vi "Freefield-Compute ASTF.vi"(0 "Stimulus":dbl[](array[numeric]), 5 "Response":dbl[](array[numeric]), 7 "Fs (Hz)":dbl=1.0, 9 "Response params":T2, 11 "error in (no error)":errorcluster) -> (6 "data":T1, 15 "error out":errorcluster)   [LabVIEW 2020]
uses:
  Common VIs/Typedefs/CAL-Response.ctl
  Common VIs/Typedefs/CAL-Data.ctl
  epl-vi-lib/Utility VIs/Math VIs/FFT x(t) to dB,Degrees (1D).vi
panel:
  out "Frequency":dbl[](array[numeric])
  out "ASTF Phase":dbl[](array[numeric])
  out "ASTF Mag":dbl[](array[numeric])
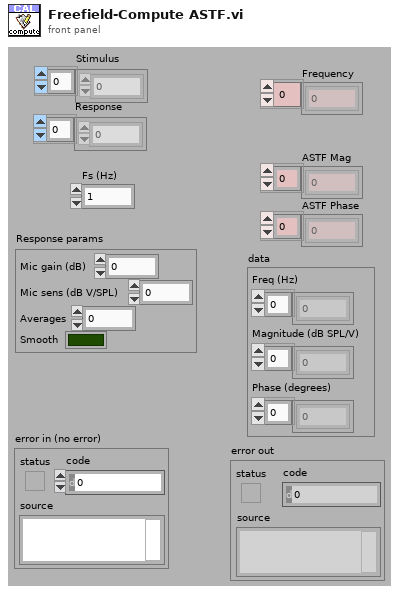
[diagram p1: front panel]
types:
  T1 = typedef "CAL-Data.ctl" = cluster{"Freq (Hz)":dbl[], "Magnitude (dB SPL/V)":dbl[], "Phase (degrees)":dbl[]}
  T2 = typedef "CAL-Response.ctl" = cluster{"Mic gain (dB)":dbl, "Mic sens (dB V/SPL)":dbl, "Averages":i32, "Smooth":bool}
  T3 = cluster{"Freq (Hz)":dbl[], "Magnitude Smoothed":dbl[], dbl[]}
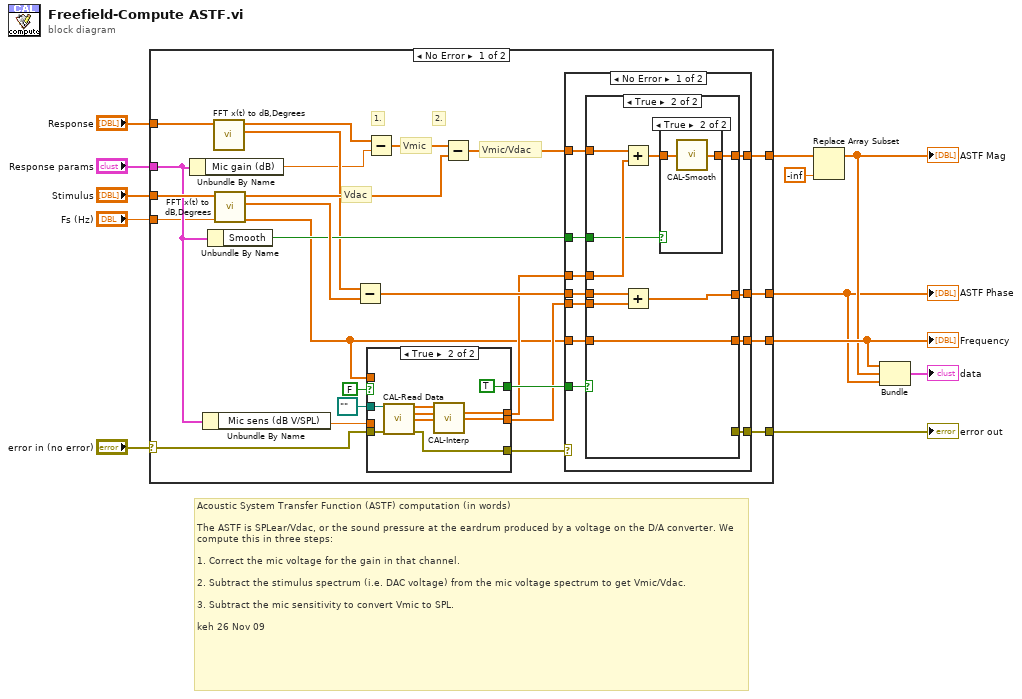
[diagram p0: block diagram]
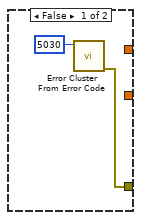
[diagram p2: hidden frame]
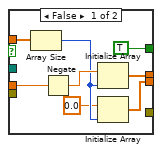
[diagram p5: hidden frame]
diagram:
  # "Acoustic System Transfer Function (ASTF) computation (in words)\n\nThe ASTF is SPLear/Vdac, or the sound pressure at the eardrum produced by a voltage on the D/A converter. We compute this in three steps:\n\n1. Correct the mic voltage for the gain in that channel.\n\n2. Subtract the stimulus spectrum (i.e. DAC voltage) from the mic voltage spectrum to get Vmic/Vdac.\n\n3. Subtract the mic sensitivity to convert Vmic to SPL.\n\nkeh 26 Nov 09"
  n1 = case shown="No Error" "error in (no error)" {
    selector: "error in (no error)" -> [w32 w82]
    tunnel: "Response" -> [w19 _]
    tunnel: [w35 _] -> w11
    tunnel: [w28 _] -> w2
    tunnel: "Stimulus" -> [w38 _]
    tunnel: [w24 _] -> w4
    tunnel: [w25 w82] -> w8
    tunnel: "Response params" -> [w14 _]
    tunnel: "Fs (Hz)" -> [w13 _]
    frame No Error {
      # "2."
      # "1."
      # "Vmic/Vdac"
      # "Vdac"
      # "Vmic"
      n2 = Unbundle By Name(w14) -> ("Mic gain (dB)"=w15:dbl)
      n3 = Unbundle By Name(w14) -> ("Mic sens (dB V/SPL)"=w31:dbl)
      n4 = Unbundle By Name(w14) -> ("Smooth"=w22:bool)
      n5 = call-poly "FFT x(t) to dB,Degrees.vi"("X"=w19) -> ("+Freq Phase of FFT (degrees)"=w17:dbl[], "+Freq. Mag of FFT (dB rms)"=w18:dbl[])  [unwired: 8 in, 1 out]
      n6 = call-poly "FFT x(t) to dB,Degrees.vi"("Fs (Hz)"=w13, "X"=w38) -> ("Freq (Hz)"=w16:dbl[], "+Freq Phase of FFT (degrees)"=w37:dbl[], "+Freq. Mag of FFT (dB rms)"=w36:dbl[])  [unwired: 7 in]
      n7 = Subtract(x=w17, y=w37) -> (x-y=w29:dbl[])
      n8 = Subtract(x=w18, y=w15) -> (x-y=w34:dbl[])
      n9 = case shown="True" FALSE {
        tunnel: w32 -> [_ w81]
        tunnel: w16 -> [w72 _]
        tunnel: path "" ("Path") -> [_ w80]
        tunnel: w31 -> [w71 _]
        tunnel: [TRUE ("arrays equal?") TRUE ("arrays equal?")] -> w27
        tunnel: [_ w79] -> w30
        tunnel: [w70 w75] -> w26
        tunnel: [w66 w74] -> w23
        frame False {
          n10 = Array Size(array=w72) -> (size(s)=w68:i32)
          n11 = Negate(x=w71) -> (-x=w69:dbl)
          n12 = Initialize Array(w69, w68) -> (w70:dbl[])
          n13 = Initialize Array(0.0 ("element"), w68) -> (w66:dbl[])
        }
        frame True {
          n14 = call "CAL-Read Data.vi"("user path"=w80, "error in (no error)"=w81) -> ("Frequency (Hz)"=w78:dbl[], "Mag"=w77:dbl[], "Phase"=w76:dbl[], "error out"=w79:errorcluster)  [unwired: 9 in, 1 out]
          n15 = call "CAL-Interp.vi"("Frequency (Hz)"=w78, "Magnitude (dB)"=w77, "Phase (degrees)"=w76) -> ("Interp Magnitude (dB)"=w75:dbl[], "Interp Phase (degrees)"=w74:dbl[])  [unwired: 9 in, 2 out]
        }
      }
      n16 = Subtract(x=w34, y=w36) -> (x-y=w33:dbl[])
      n17 = case shown="No Error" w30 {
        selector: w30 -> [_ w64]
        tunnel: w26 -> [w49 _]
        tunnel: [w48 _] -> w35
        tunnel: w33 -> [w47 _]
        tunnel: [w43 w64] -> w25
        tunnel: w29 -> [w45 _]
        tunnel: [w44 _] -> w28
        tunnel: w27 -> [w46 _]
        tunnel: w16 -> [w42 _]
        tunnel: [w41 _] -> w24
        tunnel: w23 -> [w40 _]
        tunnel: w22 -> [w39 _]
        frame No Error {
          n18 = case shown="True" w46 {
            tunnel: w49 -> [_ w60]
            tunnel: [_ w52] -> w48
            tunnel: w47 -> [_ w59]
            tunnel: w45 -> [_ w58]
            tunnel: [_ w57] -> w44
            tunnel: [w51 _] -> w43
            tunnel: w42 -> [_ w56]
            tunnel: [_ w56] -> w41
            tunnel: w40 -> [_ w55]
            tunnel: w39 -> [_ w54]
            frame False {
              n19 = call <vilib>:"Error Cluster From Error Code.vi"("error code (0)"=5030) -> ("error out"=w51:errorcluster)  [unwired: 8 in]
            }
            frame True {
              n20 = Add(x=w59, y=w60) -> (x+y=w53:dbl[])
              n21 = Add(x=w58, y=w55) -> (x+y=w57:dbl[])
              n22 = case shown="True" w54 {
                tunnel: w53 -> [w61 w63]
                tunnel: [w61 w62] -> w52
                frame False {
                }
                frame True {
                  n23 = call "CAL-Smooth.vi"("Magnitude"=w63) -> ("Magnitude Smoothed"=w62:dbl[])
                }
              }
            }
          }
        }
        frame Error {
        }
      }
    }
    frame Error {
    }
  }
  "ASTF Phase" <- w2
  "error out" <- w8
  "Frequency" <- w4
  n24 = Replace Array Subset(array=w11, new element=-inf) -> (w3:dbl[])  [unwired: 1 in]
  "ASTF Mag" <- w3
  n25 = Bundle("Freq (Hz)"=w4, "Magnitude Smoothed"=w3, w2) -> (→"data":T3)  [unwired: 1 in]
